vi "Simulation.vi"() -> ()   [LabVIEW 2016]
uses:
  Simulated DSF Custom Device/Simulated DSF Custom Device.lvclass
  C:/Git/SourceTree/DSF/Development/Testing/Simulated VeriStand Custom Device/Simulated VeriStand Custom Device.lvclass
  Simulated VeriStand Custom Device/Simulated VeriStand Custom Device.lvclass/Simulated VeriStand Custom Device.ctl
  Simulated VeriStand Engine Interface/Simulated VeriStand Engine.Interface.lvclass/Simulated VeriStand Engine.Interface.ctl
  Simulated VeriStand Engine/Simulated VeriStand Engine.lvclass/Simulated VeriStand Engine.ctl
  Simulated VeriStand Custom Device/DSF.Simulation.Custom Device.Set Channel Count.vi
  Simulated VeriStand Engine/Accessors/Simulated VeriStand Engine.Set Interface.vi
  Simulated VeriStand Engine Interface/Methods/Simulated VeriStand Engine.Interface.Create.vi
  Simulated VeriStand Engine/Accessors/Write Simulated Custom Devices.vi
  Simulated VeriStand Engine/Methods/Simulated VeriStand Engine.Allocate Channels.vi
  Simulated VeriStand Engine Interface/Methods/Simulated VeriStand Engine.Interface.Allocate.Status Pointers.vi
  Simulated VeriStand Engine Interface/Methods/Simulated VeriStand Engine.Interface.Allocate.Control Pointers.vi
  Simulated VeriStand Engine/Methods/Simulated VeriStand Engine.Get Total Channel Count.vi
  Simulated VeriStand Engine/Accessors/Write Data Ref.vi
  Source/Submodules/Memory/Source/Classes/Internal/Memory.Pointer.Internal.New.vi
  Simulated VeriStand Engine Interface/Accessors/Simulated VeriStand Engine.Interface.Set Status Pointers.vi
  Simulated VeriStand Engine Interface/Accessors/Simulated VeriStand Engine.Interface.Set Control Pointers.vi
  Simulated VeriStand Engine/Accessors/Read Simulated Custom Devices.vi
  Simulated VeriStand Custom Device/DSF.Simulation.Custom Device.Get Channel Count.vi
  Source/Submodules/Memory/Source/Classes/Internal/Memory.Pointer.Internal.Allocate.vi
  <vilib>/NI Veristand/Custom Device API/Global Data Refs.vi
  Simulated VeriStand Engine/Simulated VeriStand Engine.lvclass
  Simulated VeriStand Engine Interface/Simulated VeriStand Engine.Interface.lvclass
  Source/Submodules/Memory/Source/Classes/Internal/Memory.Pointer.Internal.lvclass
  Simulated VeriStand Custom Device/Simulated VeriStand Custom Device.lvclass
panel:
  in  "Channel Count":u32
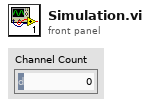
[diagram p1: front panel]
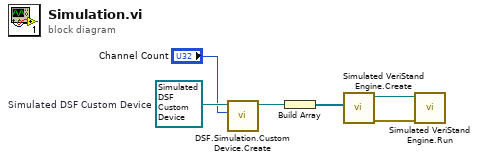
[diagram p0: block diagram]
diagram:
  w6 = refnum<class "Simulated DSF Custom Device.lvclass"> refnum  # Simulated DSF Custom Device
  n1 = call "DSF.Simulation.Custom Device.Create.vi"("Channel Count"="Channel Count", "Simulated VeriStand Custom Device in"=w6) -> ("Simulated VeriStand Custom Device out"=w4:refnum<class "Simulated DSF Custom Device.lvclass">)  [unwired: 8 in, 1 out]
  n2 = Build Array(w4) -> (w1:refnum<class "Simulated DSF Custom Device.lvclass">[])
  n3 = call "Simulated VeriStand Engine.Create.vi"("Simulated Custom Devices"=w1) -> ("error out"=w2:errorcluster, "Simulated VeriStand Engine out"=w3:refnum<class "Simulated VeriStand Engine.lvclass">)  [unwired: 9 in]
  n4 = call "Simulated VeriStand Engine.Run.vi"("error in (no error)"=w2, "Simulated VeriStand Engine in"=w3) -> ()  [unwired: 8 in, 2 out]
